vi "Close.vi"(8 "error in (no error)":errorcluster {"code" format="%.0x"}, 11 "Device ID (0)":i32) -> (0 "error out":errorcluster {"code" format="%.0x"}, 3 "Device ID out":i32)   [LabVIEW 2010, in "KEYENCE LJ-X8000A.lvlib"]
doc: "Performs an instrument error query before terminating the software connection to the instrument."
uses:
  KEYENCE LJ-X8000A.lvlib
panel:
  # "(c) 2019 KEYENCE CORPORATION.  ALL RIGHTS RESERVED."
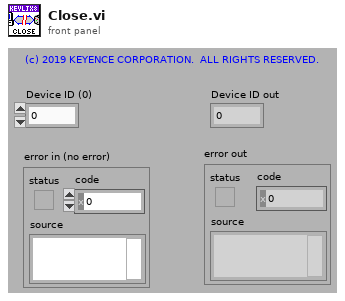
[diagram p1: front panel]
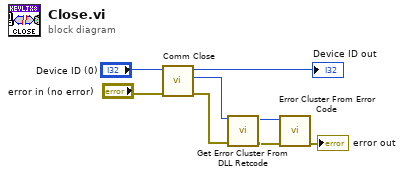
[diagram p0: block diagram]
diagram:
  n1 = call "Comm Close.vi"("error in (no error)"="error in (no error)", "Device ID (0)"="Device ID (0)") -> ("error out"=w7:errorcluster, "Return Code"=w8:i32, "Device ID out"=→"Device ID out":i32)  [unwired: 7 in]
  n2 = call "Get Error Cluster From DLL Retcode.vi"("error in (no error)"=w7, "DLL Return Code"=w8) -> ("error out"=w3:errorcluster, "VI Error Code"=w1:i32)  [unwired: 8 in]
  n3 = call <vilib>:"Error Cluster From Error Code.vi"("error in (no error)"=w3, "error code (0)"=w1) -> ("error out"=→"error out":errorcluster)  [unwired: 7 in]
